vi "BNC555.panel.vi"(0 "object ref":refnum<vi>, 5 "error in (no error)":errorcluster) -> (19 "error out":errorcluster)   [LabVIEW 2014, in "BNC555.lvlib"]
doc: "By this VI an ignitron can be monitored and switched. \n\n\"HEATING ON\" and \"WATER ON\" indicate the status (blue: bad tag value, no connection, or internal problems; lightgreen: on; red: off).\n\nThe button switches the electronic of the ignitron, \"SWITCH STATE\" indicates the switch status (blue: bad tag value, no connection, or internal problems; darkgreen: off; lightgreen: on).\n\n\"TRIGGER\" and \"TRIGGER PULSE\" indicate the status of the trigger (blue: bad tag value, no connection, or internal problems; darkgreen: off; lightgreen: on).\n\n\"on since\" indicates at which time the Ignition has been switched on.\n\n\"EXIT\" closes the front panel (GUI), while \"Delete Instance\" disconnects and removes the instance from the PCS.\n\nThis VI has no machine safety relevant logig: there is neither a check of internal conclict nor with other objects. Therefore it must be handled with care and should be operated by well educated operators only. It is forseen exclusively for direct operating and testing of the system. \n\nLicense Agreement for this software:\n\nCopyright (C)\nGesellschaft für Schwerionenforschung, GSI\nPlanckstr. 1\n64291 Darmstadt\nGermany\n\nContact: D.Beck@gsi.de \n\nThis program is free software; you can redistribute it and/or modify it under the terms of the GNU General Public License as published by the Free Software Foundation; either version 2 of the license, or (at your option) any later version.\n\nThis program is distributed in the hope that it will be useful, but WITHOUT ANYW ARRANTY; without even the implied warranty of MERCHANTABILITY or FITNESS FOR A PARTICULAR PURPOSE. See the GNU General License for more details (http://www.gnu.org).\n\nGesellschaft für Schwerionenforschung, GSI\nPlanckstr. 1, 64291 Darmstadt, Germany\nFor all questions and ideas contact: M.Richter@gsi.de, H.Brand@gsi.de or D.Beck@gsi.de.\nLast update: 18-DEC-2002"
uses:
  BNC555.lvlib
  CSPhelix/PH_StatusHandler/PH_StatusHandler.GUI element.ctl
  non_GPL/instr.lib/BNC555/BNC555_U.llb/BNC555 All Chan Parameters.ctl
  non_GPL/instr.lib/BNC555/BNC555_U.llb/BNC555 All Sys Parameters.ctl
  CSCore/CSObj/CSObj.lvlib
  CSPhelix/PH_Common/PH_Common.lvlib
  CSPhelix/PH_Class/PH_Class.lvlib
  CSPhelix/PH_PSDBWriter/PH_PSDBWriter.lvlib
  CSPhelix/PH_StatusHandler/PH_StatusHandler.lvlib
  non_GPL/instr.lib/BNC555/BNC555 - Driver np.lvlib
panel:
  out "PSDB Status":u32(colorbox)=6618880 caption="PSDB"
  out "Instr Option":string
  out "Instr Firmware Revision":string
  out "Instr Driver Revision":string
  out "Self-Test Response":string
  out "Device Error":errorcluster
  out "System":T1={"Sys Period"=0.0, "Sys Oscillator"=FALSE, "Sys Mode"=enum."Normal", "Sys Burst #"=0, "Sys DC On"=10, "Sys DC Off"=5, "Sys Trig Mode"=enum."Gated", "Sys Trig Lev"=2.5, "Sys Gate State"=TRUE, "Sys Trig Edge"=TRUE, "Sys State"=TRUE} {"Sys Period" format="%.6p"; "Sys Trig Lev" format="%.4p"}
  out "Channel Array":T2[](array[typedef]) {"Chan Lev Adjust" format="%.3p"; "Chan Width" format="%.3p"; "Chan Delay" format="%.3p"; "Chan #" items=["System (To)", "Channel A", "Channel B", "Channel C", "Channel D", "Channel E", "Channel F", "Channel G", "Channel H"]}
  out "Information":T3={"VISA resource name"="", "Baud Rate (1:9600)"=1} {"Baud Rate (1:9600)" items=["4800", "9600", "19200", "38400"]}
  out "Status":T4 caption="Enabling State"
  in  "Delete":bool
  in  "Exit":bool
  # "PCS"
  # "3.40"
  # "Run\nStop"
  # "System (To) Mode"
  # "Triggering"
  # "High\nLow"
  # "Rising\nFalling"
  # "External\nInternal"
  # "Output"
  # "Gate"
  # "On\nOff"
  # "Pulse"
  # "On\nOff"
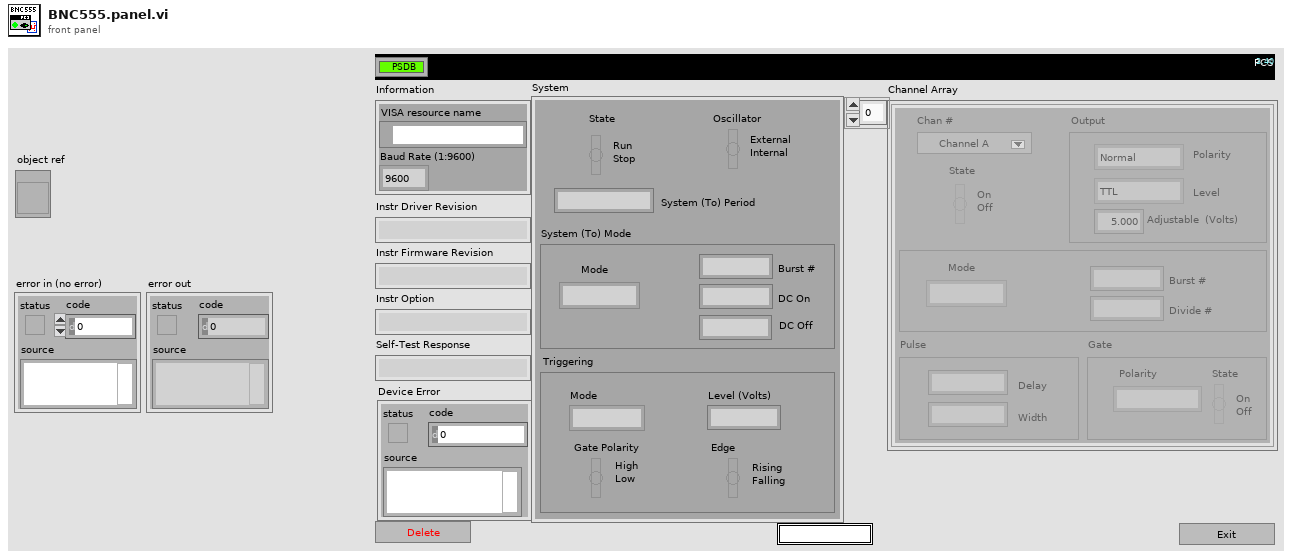
[diagram p1: front panel]
types:
  T1 = typedef "BNC555 - Driver np.lvlib/BNC555 All Sys Parameters.ctl" = cluster{"Sys Period":dbl, "Sys Oscillator":bool, "Sys Mode":enum16{"Normal", "Single", "Burst", "Duty Cycle"}, "Sys Burst #":u32, "Sys DC On":u32, "Sys DC Off":u32, "Sys Trig Mode":enum16{"Disabled", "Triggered", "Gated"}, "Sys Trig Lev":dbl, "Sys Gate State":bool, "Sys Trig Edge":bool, "Sys State":bool}
  T2 = typedef "BNC555 - Driver np.lvlib/BNC555 All Chan Parameters.ctl" = cluster{"Chan #":i32, "Chan State":bool, "Chan Delay":dbl, "Chan Width":dbl, "Chan Mode":enum16{"Normal", "Single", "Burst", "Divide by N"}, "Chan Burst #":u32, "Chan Divide #":u32, "Chan Pol Out":enum16{"Normal", "Complement", "Inverted"}, "Chan Level Out":enum16{"TTL", "Adjustable", "35 Volt"}, "Chan Lev Adjust":dbl, "Chan Gate Pol":enum16{"Normal", "Complement", "Inverted"}, "Chan Gate State":bool}
  T3 = cluster{"VISA resource name":refnum<visa-resource-name>, "Baud Rate (1:9600)":u16}
  T4 = typedef "PH_StatusHandler.lvlib/PH_StatusHandler.GUI element.ctl" = u16
  T5 = typedef "BNC555.lvlib/BNC555.i attribute.ctl" = cluster{"Information":cluster{"VISA resource name":refnum<visa-resource-name>, "Baud Rate (1:9600)":u16}, "Channel Array":T2[], "System":T1, "GUI Refs":cluster{"Delete":refnum<vi>, "Information":refnum<vi>, "System":refnum<vi>, "Channel Array":refnum<vi>, "Device Error":refnum<vi>, "Instr Driver Revision":refnum<vi>, "Instr Firmware Revision":refnum<vi>, "Instr Option":refnum<vi>, "Self-Test Response":refnum<vi>}, "Service IDs Channelinfo":i32[], "Service ID T0 Mode":i32}
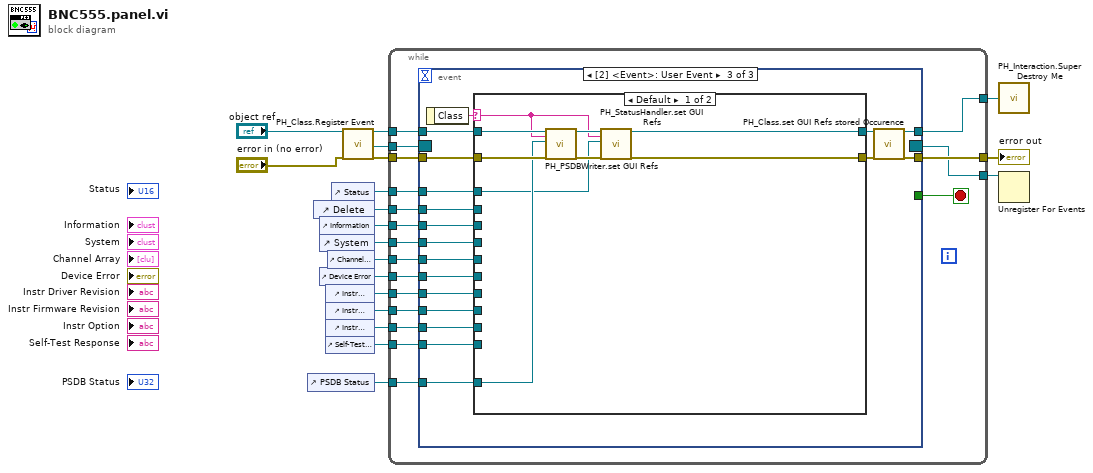
[diagram p0: block diagram]
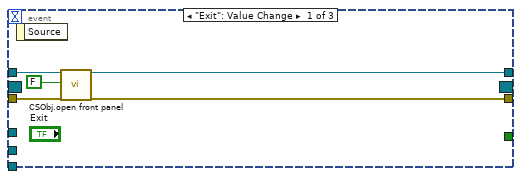
[diagram p2: hidden frame]
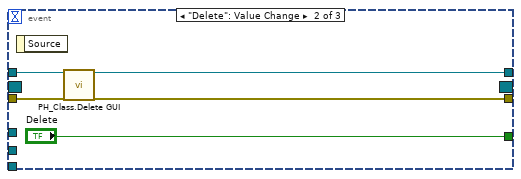
[diagram p3: hidden frame]
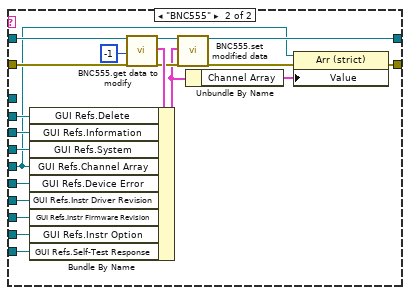
[diagram p4: hidden frame]
diagram:
  n1 = control-ref of="PSDB Status"() -> (w11:refnum<vi>)
  n2 = control-ref of="Delete"() -> (w10:refnum<vi>)
  n3 = control-ref of="Information"() -> (w9:refnum<vi>)
  n4 = control-ref of="System"() -> (w8:refnum<vi>)
  n5 = control-ref of="Device Error"() -> (w6:refnum<vi>)
  n6 = control-ref of="Instr Driver Revision"() -> (w5:refnum<vi>)
  n7 = control-ref of="Instr Firmware Revision"() -> (w4:refnum<vi>)
  n8 = control-ref of="Instr Option"() -> (w3:refnum<vi>)
  n9 = control-ref of="Self-Test Response"() -> (w2:refnum<vi>)
  n10 = control-ref of="Channel Array"() -> (w7:refnum<vi>)
  n11 = control-ref of="Status"() -> (w1:refnum<vi>)
  n12 = call "PH_Class.Register Event.vi"("i ref in"="object ref", "error in (no error)"="error in (no error)") -> ("i ref out"=w17:refnum<vi>, "Event Registration Refnum"=w15:refnum<event-registration>, "error out"=w16:errorcluster)  [unwired: 15 in]
  n13 = while {
    tunnel: w17 -> [w34]
    tunnel: [w33] -> w19
    tunnel: w16 -> [w36]
    tunnel: [w35] -> w18
    tunnel: w15 -> [w32]
    tunnel: [w31] -> w14
    tunnel: w11 -> [w30]
    tunnel: w10 -> [w29]
    tunnel: w1 -> [w28]
    tunnel: w9 -> [w27]
    tunnel: w8 -> [w26]
    tunnel: w7 -> [w25]
    tunnel: w6 -> [w24]
    tunnel: w5 -> [w23]
    tunnel: w4 -> [w22]
    tunnel: w3 -> [w21]
    tunnel: w2 -> [w20]
    stop <- w37 stop-if-true
    n14 = event shown="[2] <Event>: User Event" {
      selector: w32 -> [_ _ _]
      dyn-events: [_ _ _] -> w31
      timeout: _ -> [_ _ _]
      tunnel: [_ "Delete" _] -> w37
      tunnel: w34 -> [w42 w46 w65]
      tunnel: w36 -> [w40 w45 w64]
      tunnel: [w39 w44 w60] -> w35
      tunnel: [w38 w43 w62] -> w33
      tunnel: w30 -> [_ _ w58]
      tunnel: w29 -> [_ _ w57]
      tunnel: w28 -> [_ _ w56]
      tunnel: w27 -> [_ _ w55]
      tunnel: w26 -> [_ _ w54]
      tunnel: w25 -> [_ _ w53]
      tunnel: w24 -> [_ _ w52]
      tunnel: w23 -> [_ _ w51]
      tunnel: w22 -> [_ _ w50]
      tunnel: w21 -> [_ _ w49]
      tunnel: w20 -> [_ _ w48]
      event "Exit": Value Change {
        n15 = event-data() -> ()  [unwired: 1 in, 1 out]
        n16 = call "CSObj.open front panel.vi"("i ref in"=w42, "frontPanelOpen"=FALSE ("front panel open"), "error in (no error)"=w40) -> ("i ref out"=w38:refnum<vi>, "error out"=w39:errorcluster)  [unwired: 15 in]
      }
      event "Delete": Value Change {
        n17 = event-data() -> ()  [unwired: 1 in, 1 out]
        n18 = call "PH_Class.Delete GUI.vi"("VI in"=w46, "error in (no error)"=w45) -> ("VI out"=w43:refnum<vi>, "error out"=w44:errorcluster)  [unwired: 16 in]
      }
      event User Event {
        n19 = event-data() -> ("Class"=w59:string)  [unwired: 1 in]
        n20 = case shown="Default" w59 {
          selector: w59 -> [w67 _]
          tunnel: w65 -> [w74 w90]
          tunnel: w64 -> [w73 w89]
          tunnel: [w68 w88] -> w63
          tunnel: [w70 w78] -> w61
          tunnel: w58 -> [w71 _]
          tunnel: w57 -> [_ w87]
          tunnel: w56 -> [w66 _]
          tunnel: w55 -> [_ w86]
          tunnel: w54 -> [_ w85]
          tunnel: w53 -> [_ w75]
          tunnel: w52 -> [_ w84]
          tunnel: w51 -> [_ w83]
          tunnel: w50 -> [_ w82]
          tunnel: w49 -> [_ w81]
          tunnel: w48 -> [_ w80]
          frame Default {
            n21 = call "PH_PSDBWriter.set GUI Refs.vi"("i ref in"=w74, "Class"=w67, "Ref PSDB Status"=w71, "error in"=w73) -> ("i ref out"=w69:refnum<vi>, "error out"=w72:errorcluster)  [unwired: 14 in]
            n22 = call "PH_StatusHandler.set GUI Refs.vi"("i ref in"=w69, "Class"=w67, "GUI Ref"=w66, "error in (no error)"=w72) -> ("i ref out"=w68:refnum<vi>, "error out"=w70:errorcluster)  [unwired: 14 in]
          }
          frame "BNC555" {
            n23 = call "BNC555.get data to modify.vi"("i ref in"=w90, "ms timeout (10000)"=-1, "error in (no error)"=w89) -> ("i ref out"=w91:refnum<vi>, "i attribute"=w93:T5, "error out"=w92:errorcluster)  [unwired: 13 in, 1 out]
            n24 = Bundle By Name(cluster=w93, "GUI Refs.Delete"=w87, "GUI Refs.Information"=w86, "GUI Refs.System"=w85, "GUI Refs.Channel Array"=w75, "GUI Refs.Device Error"=w84, "GUI Refs.Instr Driver Revision"=w83, "GUI Refs.Instr Firmware Revision"=w82, "GUI Refs.Instr Option"=w81, "GUI Refs.Self-Test Response"=w80) -> (w77:T5)
            n25 = call "BNC555.set modified data.vi"("i ref in"=w91, "i attribute"=w77, "error in (no error)"=w92) -> ("i ref out"=w88:refnum<vi>, "error out"=w79:errorcluster)  [unwired: 15 in]
            n26 = Unbundle By Name(w77) -> ("Channel Array"=w76:T2[])
            n27 = property class="Arr (strict)"(reference=w75, error in=w79, "Value"=w76) -> (error out=w78:errorcluster)  [unwired: 1 out]
          }
        }
        n28 = call "PH_Class.set GUI Refs stored Occurence.vi"("i ref in"=w63, "error in (no error)"=w61) -> ("i ref out"=w62:refnum<vi>, "error out"=w60:errorcluster)  [unwired: 16 in]
      }
    }
  }
  "error out" <- w18
  n29 = call "PH_Interaction.Super Destroy Me.vi"("i ref out"=w19) -> ()
  n30 = Unregister For Events(event registration refnum=w14) -> ()  [unwired: 1 in, 1 out]
